vi "RB2 parse navigation string.vi"(2 "Header":string="G", 3 "Nav String":string="$,G,274,67,B,245,67,R,255,42,N,282,44,S,14,5,395\r") -> (0 "Valid?":bool, 1 "Jeep Data":cluster{"Header":string, i32, i32})   [LabVIEW 2012]
doc: "This VI will parse the Tug navigation string for the Tug letters, A for example, and the time, T. It returns a cluster with the Tug / Time and three values as decimals."
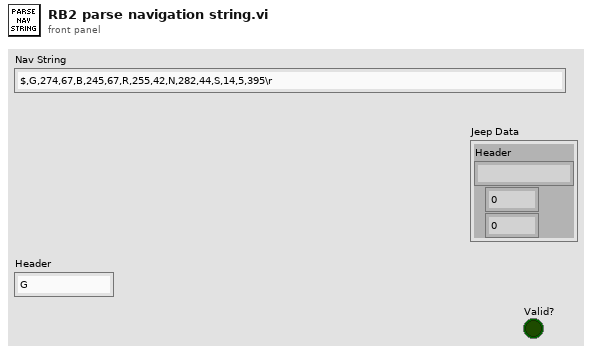
[diagram p1: front panel]
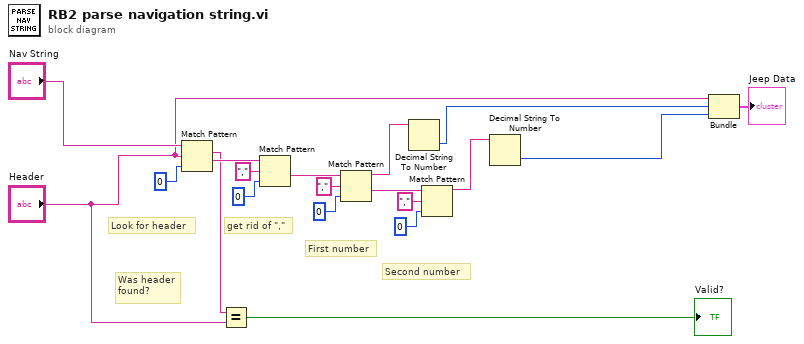
[diagram p0: block diagram]
diagram:
  # "Was header\nfound?"
  # "Second number"
  # "First number"
  # "get rid of \",\""
  # "Look for header"
  n1 = Match Pattern(string="Nav String", regular expression="Header", offset (0)=0) -> (match substring=w5:string, after substring=w8:string)  [unwired: 2 out]
  n2 = Equal?(x=w5, y="Header") -> (x = y?=→"Valid?":bool)
  n3 = Match Pattern(string=w8, regular expression=",", offset (0)=0) -> (after substring=w9:string)  [unwired: 3 out]
  n4 = Match Pattern(string=w9, regular expression=",", offset (0)=0) -> (before substring=w16:string, after substring=w12:string)  [unwired: 2 out]
  n5 = Decimal String To Number(string=w16) -> (number=w7:i32)  [unwired: 2 in, 1 out]
  n6 = Match Pattern(string=w12, regular expression=",", offset (0)=0) -> (before substring=w13:string)  [unwired: 3 out]
  n7 = Decimal String To Number(string=w13) -> (number=w2:i32)  [unwired: 2 in, 1 out]
  n8 = Bundle("Header"="Header", w7, w2) -> (→"Jeep Data":cluster{"Header":string, i32, i32})  [unwired: 1 in]
